vi "to_json.vi"(8 "error in":errorcluster, 11 "timestampMetadata in":refnum<class "timestampMetadata.lvclass">) -> (0 "error out":errorcluster, 2 "json":string, 3 "timestampMetadata out":refnum<class "timestampMetadata.lvclass">, 4 "Not Default":bool)   [LabVIEW 2020, in "timestampMetadata.lvclass"]
uses:
  timestampMetadata.lvclass
  timestampType/timestampType.lvclass
  timestampMetadata.lvclass/timestampMetadata.ctl
  f81aad97-b53f-4cee-8283-f8a4a184eeeb.vi
  <vilib>/JDP Science/JSONtext/Variant to JSON Text.vi
  <vilib>/JDP Science/JSONtext/support/Format JSON Object.vi
  <vilib>/JDP Science/JSONtext/LVClass Serializer/JSONtext LVClass Serializer.lvclass
  <vilib>/JDP Science/JSONtext/JSONtext.lvlib
  5594e85e-0340-4586-878d-f84de8e7955c.vi
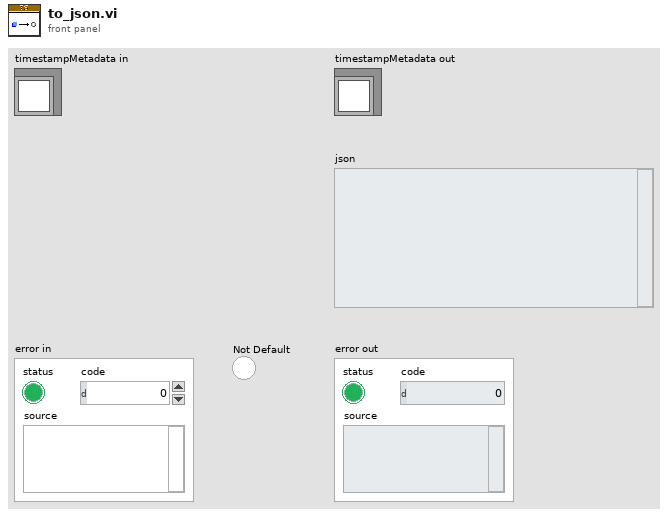
[diagram p1: front panel]
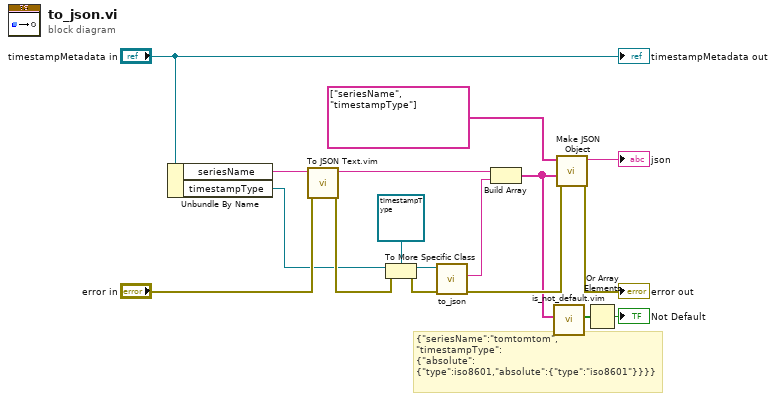
[diagram p0: block diagram]
diagram:
  # "{\"seriesName\":\"tomtomtom\",\n\"timestampType\":\n{\"absolute\":\n{\"type\":iso8601,\"absolute\":{\"type\":\"iso8601\"}}}}"
  n1 = Unbundle By Name("timestampMetadata in") -> ("seriesName"=w12:string, "timestampType"=w4:refnum<class "timestampType.lvclass">)
  n2 = call "To JSON Text.vim"("error in (no error)"="error in", "Anything"=w12) -> ("error out"=w5:errorcluster, "<JSON>"=w16:string)  [unwired: 8 in]
  n3 = To More Specific Class(target class=refnum<class "timestampType.lvclass"> refnum ("timestampType"), reference=w4, error in=w5) -> (specific class reference=w11:refnum<class "timestampType.lvclass">, error out=w10:errorcluster)
  n4 = call-dynamic "to_json.vi"("error in"=w10, "timestampType in"=w11) -> ("error out"=w8:errorcluster, "json"=w7:string)  [unwired: 6 in, 2 out]
  n5 = Build Array(w16, w7) -> (w2:string[])
  n6 = call "is_not_default.vim"("data"=w2) -> ("Not Default"=w3:bool[])  [unwired: 10 in]
  n7 = call <vilib>:"Make JSON Object.vi"("error in (no error)"=w8, "JSON Items"=w2, "Item Names"=string[] ["seriesName", "timestampType"]) -> ("error out"=→"error out":errorcluster, "<JSON>"=→"json":string)  [unwired: 7 in]
  n8 = Or Array Elements(Boolean array=w3) -> (logical OR=→"Not Default":bool)
  "timestampMetadata out" <- "timestampMetadata in"
